vi "Agilent34410A Set Function.vi"(8 "error in (no error)":errorcluster, 10 "DMM Function":T1, 11 "VISA Rsrc":refnum<visa-resource-name>="SR530") -> (0 "error out":errorcluster, 3 "VISA Rsrc Out":refnum<visa-resource-name>="GPIB0::12::INSTR", 4 "ChaineCom":string caption="Chaîne de commande")   [LabVIEW 2019]
uses:
  <userlib>/Agilent34410A/Agilent34410A DMM_Func.ctl
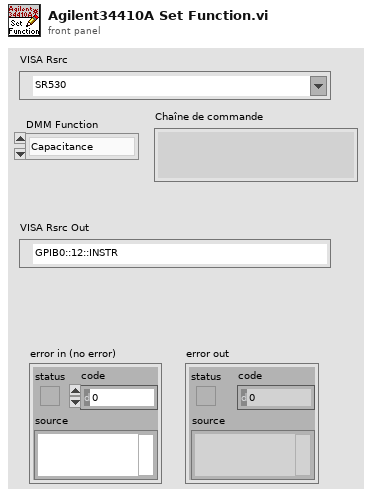
[diagram p1: front panel]
types:
  T1 = typedef "Agilent34410A DMM_Func.ctl" = enum16{"Capacitance", "Continuity", "Current AC", "Current", "Diode", "Frequency", "4W Resistance", "Period", "Resistance", "Temperature", "Voltage AC", "Voltage"}
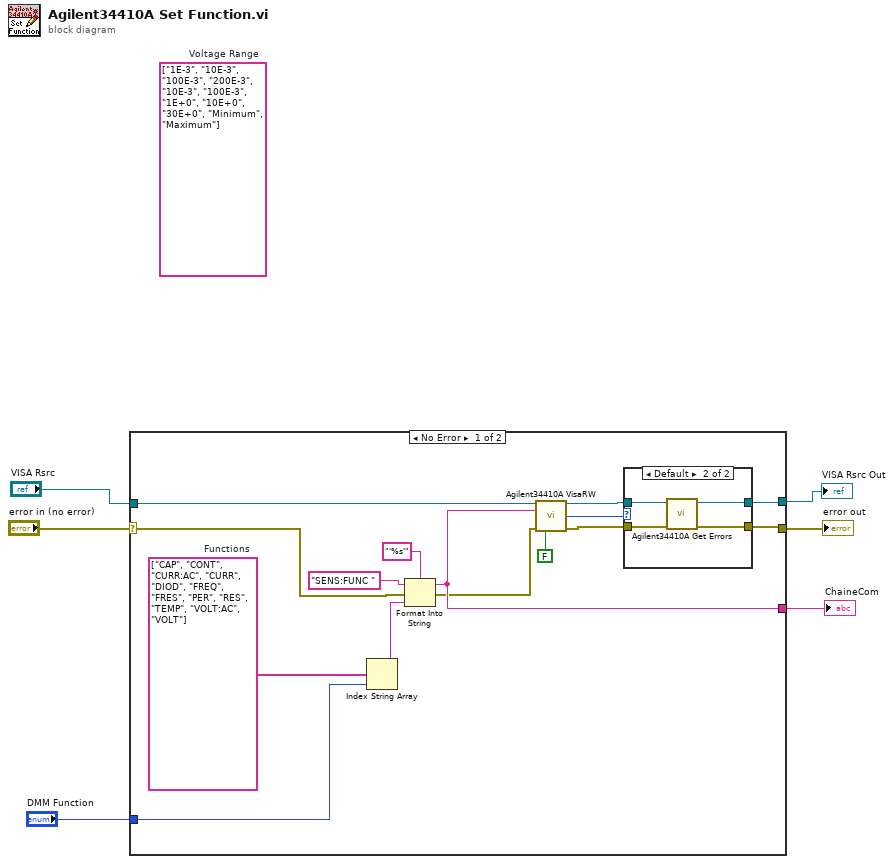
[diagram p0: block diagram]
diagram:
  (unwired) string[] ["1E-3", "10E-3", "100E-3", "200E-3", "10E-3", "100E-3", "1E+0", "10E+0", "30E+0", "Minimum", "Maximum"]  # Voltage Range
  n1 = case shown="No Error" "error in (no error)" {
    selector: "error in (no error)" -> [w14 w28]
    tunnel: "VISA Rsrc" -> [w21 w29]
    tunnel: [w8 w28] -> w4
    tunnel: [w7 w29] -> w3
    tunnel: [w15 _] -> w2
    tunnel: "DMM Function" -> [w12 _]
    frame No Error {
      w20 = string[] ["CAP", "CONT", "CURR:AC", "CURR", "DIOD", "FREQ", "FRES", "PER", "RES", "TEMP", "VOLT:AC", "VOLT"]  # Functions
      n2 = Index String Array(1:w12, 2:w20) -> (0:w18:string)  [unwired: 1 in]
      n3 = Format Into String(format string="'%s'" ("string (\"\")"), initial string="SENS:FUNC " ("string (\"\")"), error in=w14, w18) -> (resulting string=w15:string, error out=w13:errorcluster)
      n4 = call <userlib>:"Agilent34410A VisaRW.vi"("VISA Rsrc"=w21, "ChaineCom"=w15, "error in (no error)"=w13, "Lecture?(T)"=FALSE) -> ("VISA Rsrc Out"=w11:refnum<visa-resource-name>, "octet d'état"=w10:u16, "error out"=w9:errorcluster)  [unwired: 7 in, 2 out]
      n5 = case shown="Default" w10 {
        tunnel: w11 -> [w23 w27]
        tunnel: w9 -> [w22 w26]
        tunnel: [w22 w25] -> w8
        tunnel: [w23 w24] -> w7
        frame 0 {
        }
        frame Default {
          n6 = call <userlib>:"Agilent34410A Get Errors.vi"("error in (no error)"=w26, "VISA Rsrc"=w27) -> ("error out"=w25:errorcluster, "VISA Rsrc Out"=w24:refnum<visa-resource-name>)  [unwired: 7 in, 1 out]
        }
      }
    }
    frame Error {
    }
  }
  "error out" <- w4
  "VISA Rsrc Out" <- w3
  "ChaineCom" <- w2
